vi "记录字符串解析到数组表.vi"(9 "导出条件":T1, 10 "记录数据":T9, 11 "名称":string) -> (0 "累积列表-标题行":string[](array[string])=["名称", "起始时间", "结束时间", "时长", "累积", "平均"], 1 "报警列表-标题行":string[](array[string])=["名称", "起始时间", "类型", "时长", "平均值", "最大值", "累积", "结论"], 2 "报警列表数组":string[][](array[string]), 3 "累积记录数组":string[][](array[string]))   [LabVIEW 2017]
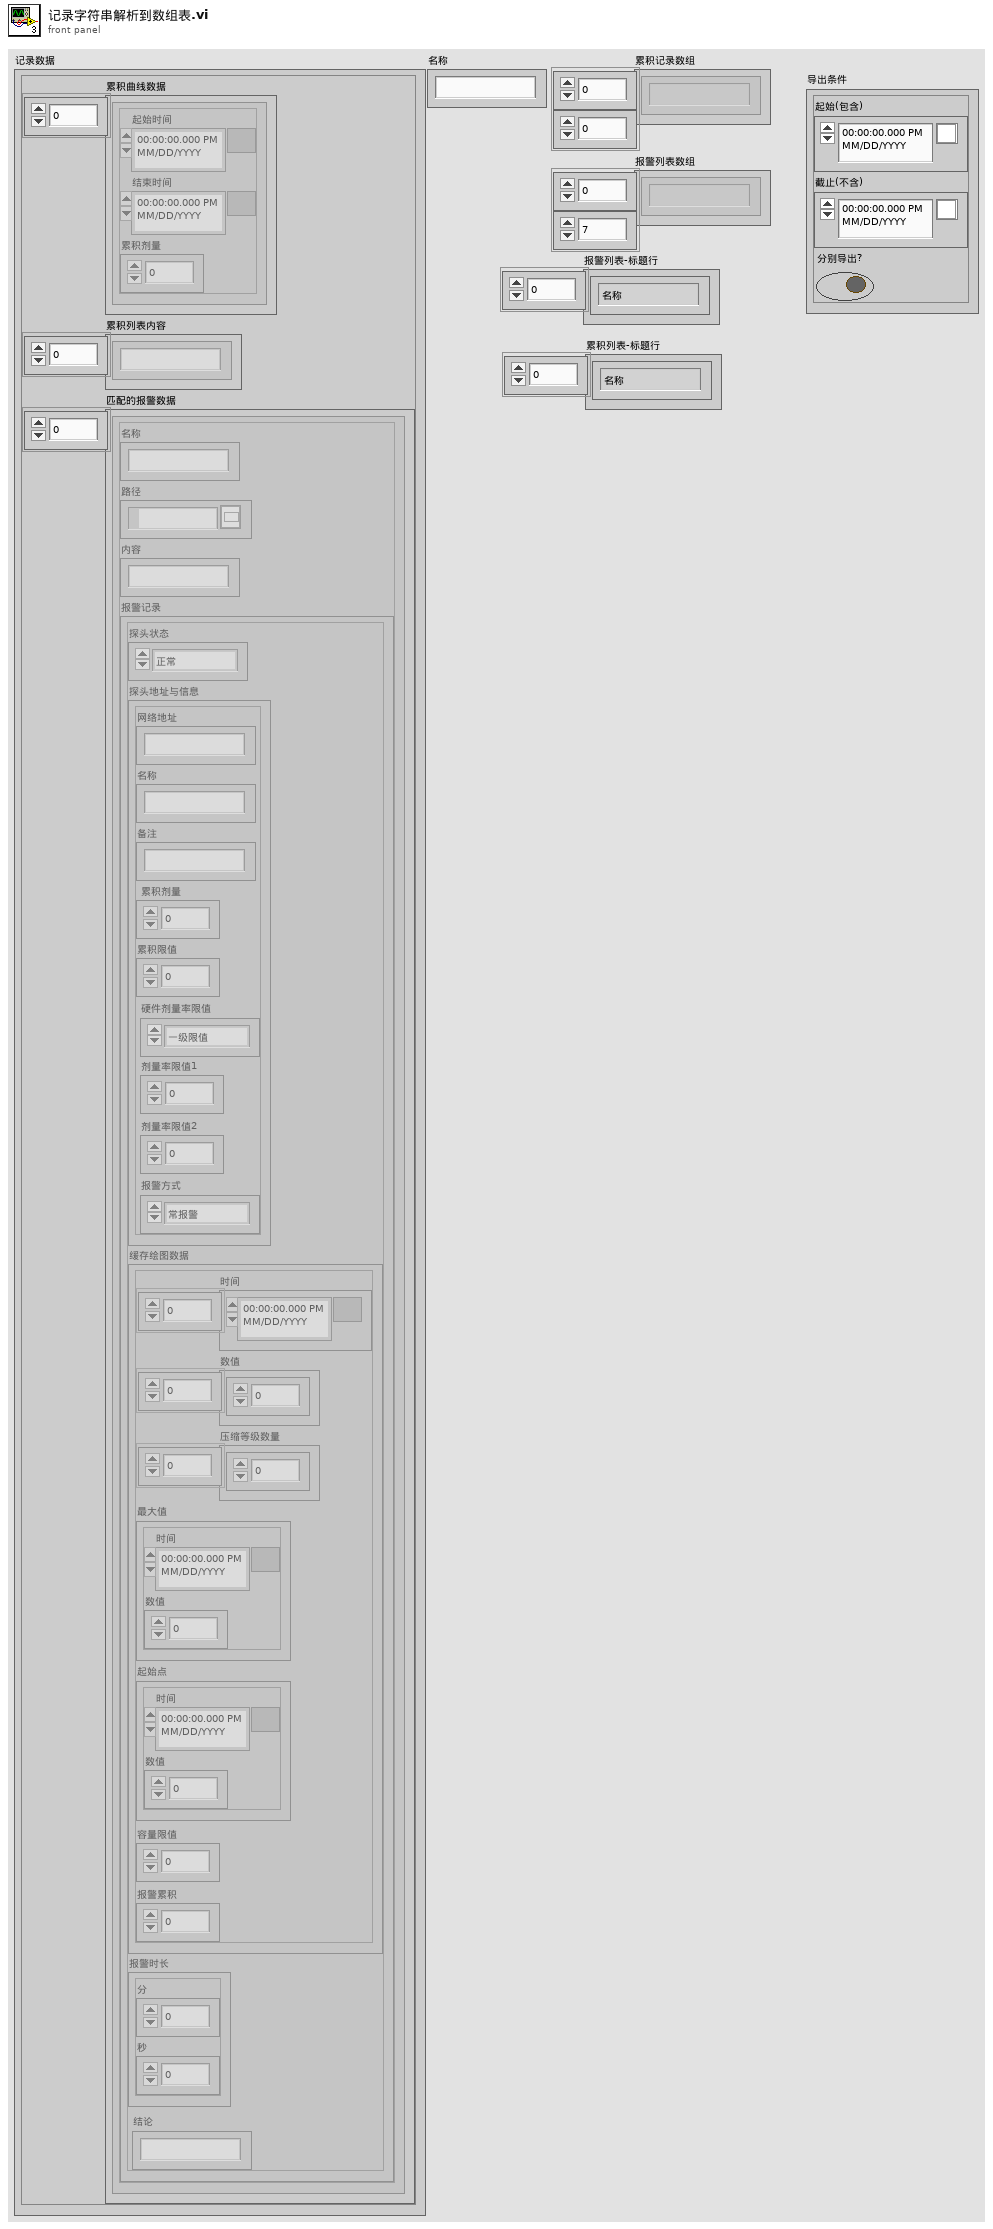
[diagram p1: front panel]
types:
  T1 = typedef "文件导出条件.ctl" = cluster{"起始(包含)":timestamp, "截止(不含)":timestamp, "分别导出?":bool}
  T2 = typedef "单条累积记录.ctl" = cluster{"起始时间":timestamp, "结束时间":timestamp, "累积剂量":dbl}
  T3 = typedef "通用报警记录.ctl" = cluster{"探头状态":T4, "探头地址与信息":T5, "缓存绘图数据":T8, "平均值":dbl, "报警时长":cluster{"分":u16, "秒":u16}, "结论":string}
  T4 = typedef "探头状态.ctl" = enum16{"正常", "离线", "禁用", "一级报警", "二级报警", "累积报警"}
  T5 = typedef "探测器信息.ctl" = cluster{"网络地址":string, "名称":string, "备注":string, "累积剂量":dbl, "累积限值":dbl, "硬件剂量率限值":T6, "剂量率限值1":dbl, "剂量率限值2":dbl, "报警方式":T7}
  T6 = typedef "探头剂量率限值选择.ctl" = enum16{"一级限值", "二级限值"}
  T7 = typedef "报警方式选择.ctl" = enum16{"常报警", "自动静音", "手动静音"}
  T8 = typedef "时值缓存压缩模块.lvlib/缓存数据.ctl" = cluster{"时间":timestamp[], "数值":dbl[], "压缩等级数量":i32[], "最大值":cluster{"时间":timestamp, "数值":dbl}, "起始点":cluster{"时间":timestamp, "数值":dbl}, "容量限值":i32, "报警累积":dbl}
  T9 = cluster{"累积曲线数据":T2[], "累积列表内容":string[], "匹配的报警数据":cluster{"名称":string, "路径":path, "内容":string, "报警记录":T3}[]}
  T10 = cluster{"名称":string, "路径":path, "内容":string, "报警记录":T3}[]
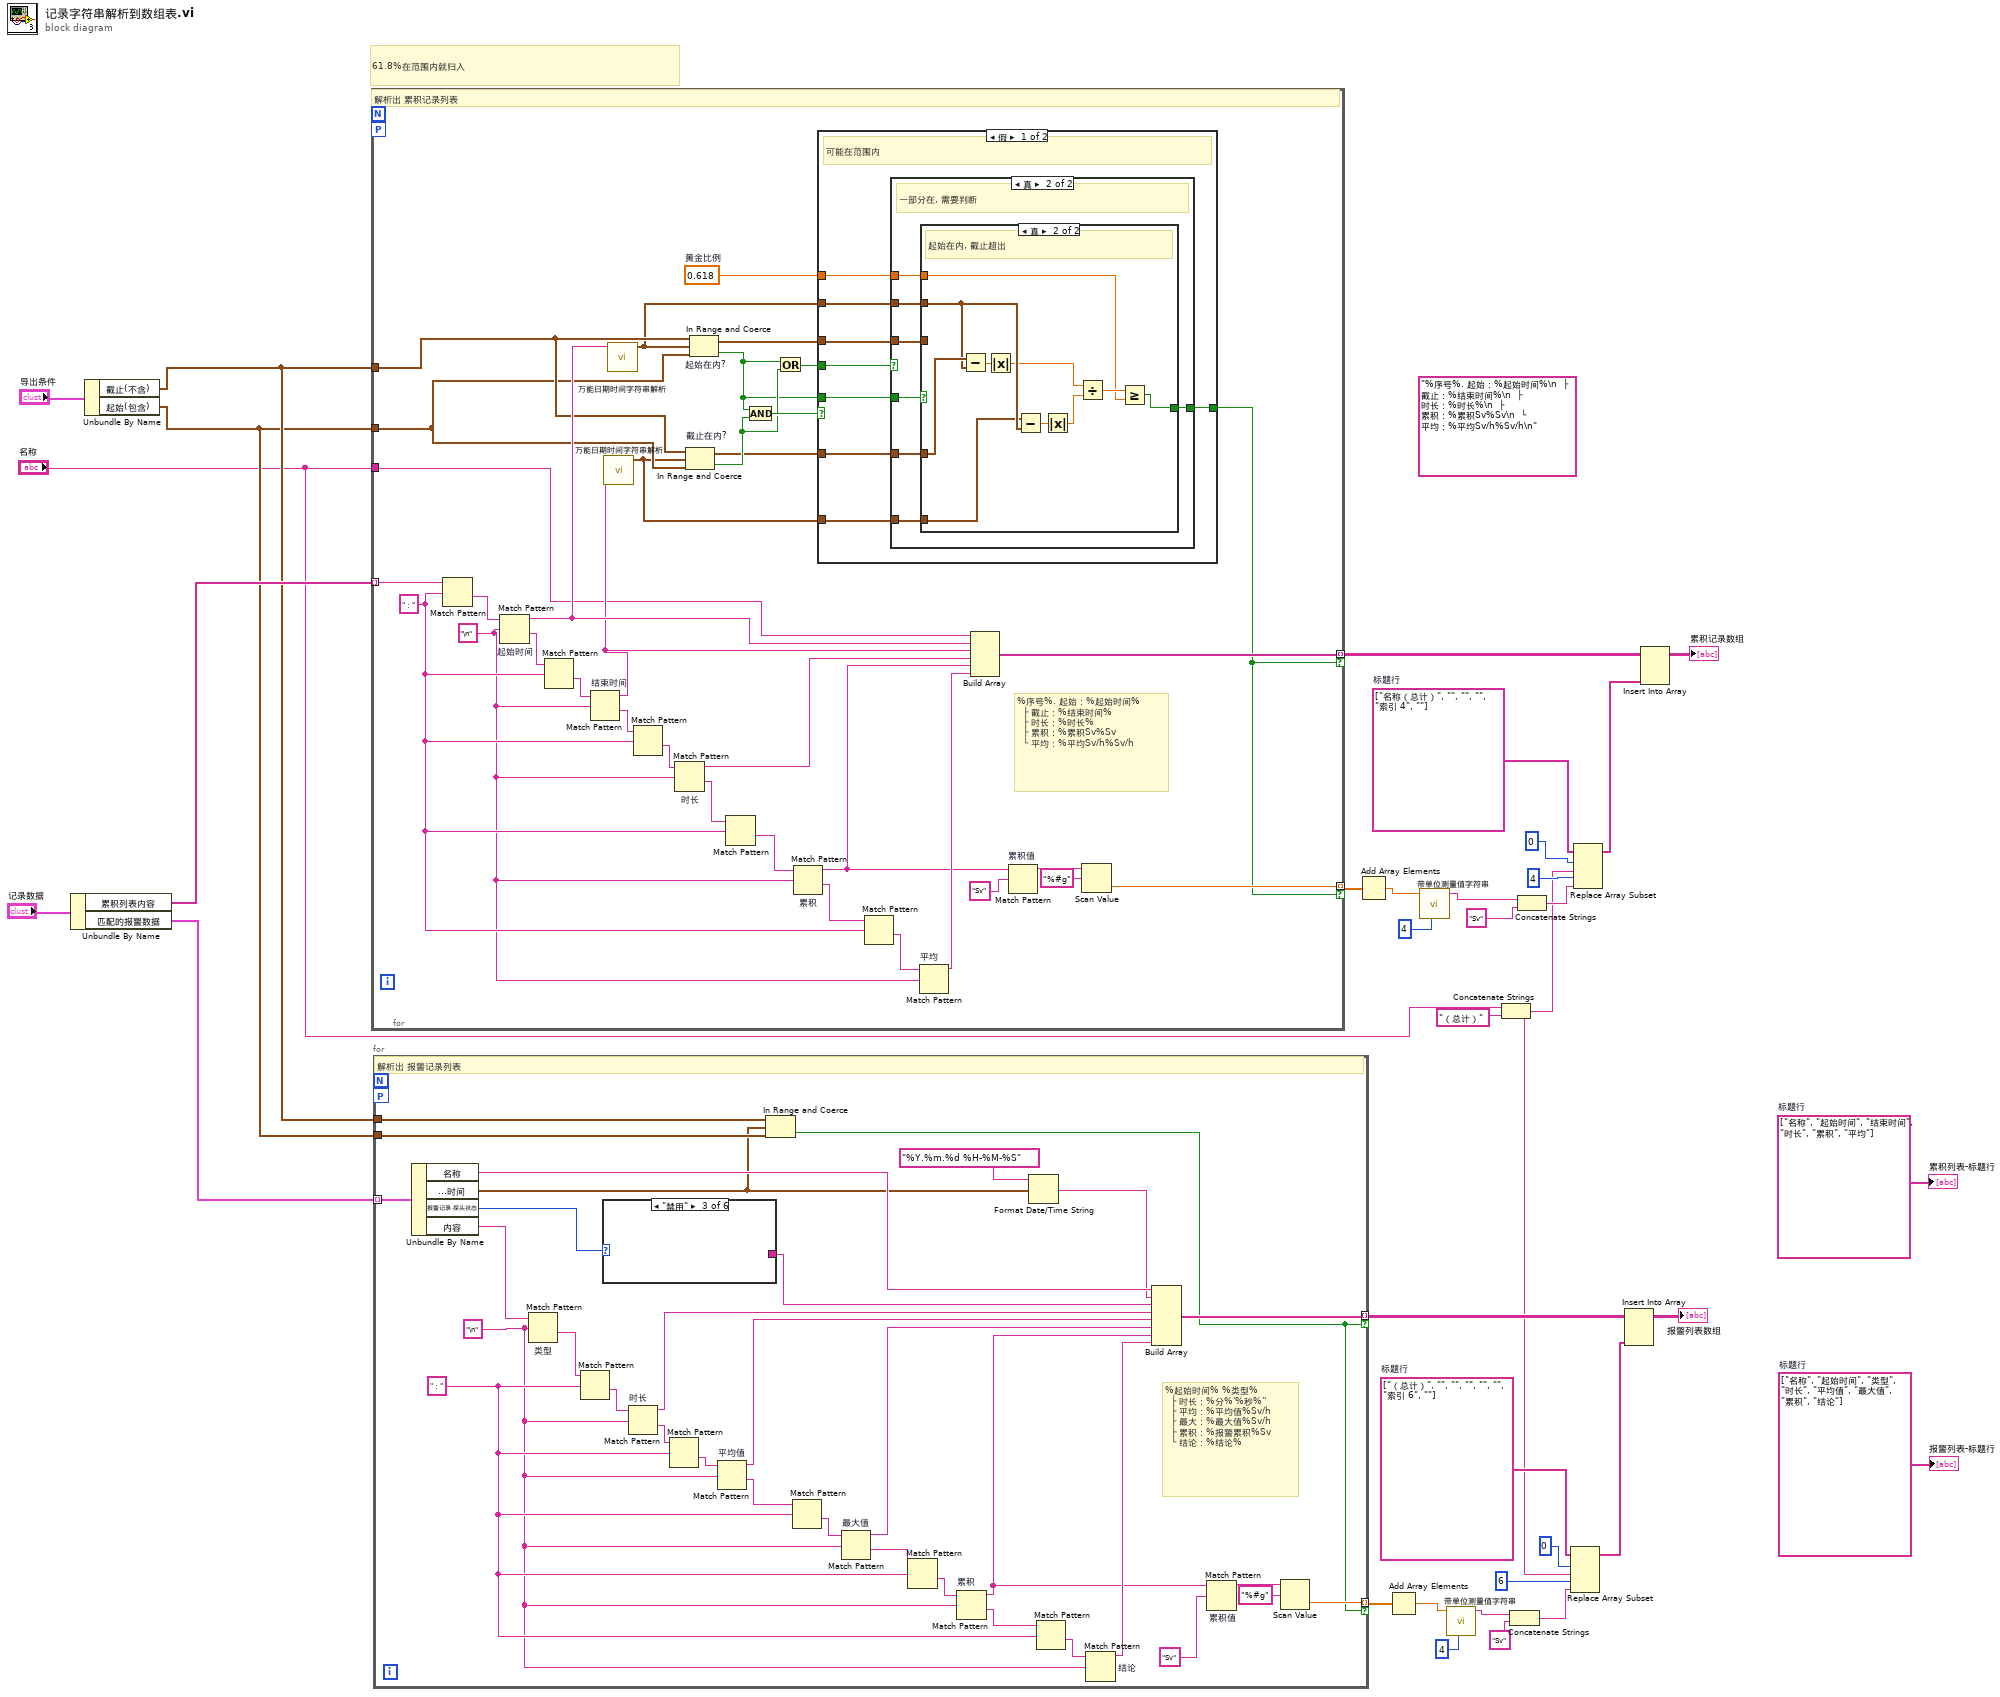
[diagram p0: block diagram]
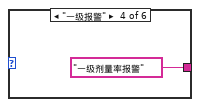
[diagram p4: hidden frame]
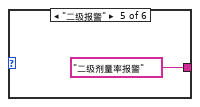
[diagram p5: hidden frame]
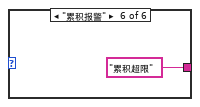
[diagram p6: hidden frame]
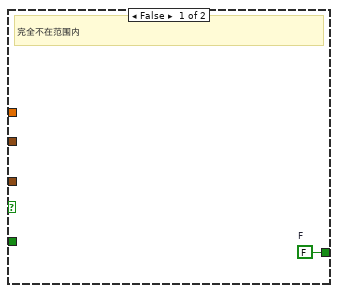
[diagram p7: hidden frame]
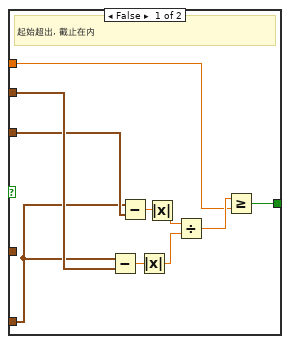
[diagram p8: hidden frame]
diagram:
  w25 = string[] ["（总计）", "", "", "", "", "", "索引 6", ""]  # 标题行
  w17 = string[] ["名称（总计）", "", "", "", "索引 4", ""]  # 标题行
  (unwired) "%序号%. 起始：%起始时间%\n  ├ 截止：%结束时间%\n  ├ 时长：%时长%\n  ├ 累积：%累积Sv%Sv\n  └ 平均：%平均Sv/h%Sv/h\n" ("Result")
  w32 = string[] ["名称", "起始时间", "类型", "时长", "平均值", "最大值", "累积", "结论"]  # 标题行
  w31 = string[] ["名称", "起始时间", "结束时间", "时长", "累积", "平均"]  # 标题行
  # "61.8%在范围内就归入"
  n1 = Unbundle By Name("记录数据") -> ("累积列表内容"=w34:string[], "匹配的报警数据"=w33:T10)
  n2 = Unbundle By Name("导出条件") -> ("截止(不含)"=w29:timestamp, "起始(包含)"=w28:timestamp)
  n3 = for {
    tunnel: w34 -> [w70] mode=indexing
    tunnel: "名称" -> [w51]
    tunnel: [w56] -> w14 mode=indexing if=w36
    tunnel: w29 -> [w53]
    tunnel: w28 -> [w52]
    workers-P: _ -> [_]
    tunnel: [w37] -> w27 mode=indexing if=w36
    w42 = 0.618  # 黄金比例
    w65 = "\n"
    w66 = "：" ("正则表达式")
    # "%序号%. 起始：%起始时间%\n  ├ 截止：%结束时间%\n  ├ 时长：%时长%\n  ├ 累积：%累积Sv%Sv\n  └ 平均：%平均Sv/h%Sv/h"
    # "解析出 累积记录列表"
    n4 = Match Pattern(string=w70, regular expression=w66) -> (after substring=w69:string)  [unwired: 1 in, 3 out]
    n5 = Match Pattern "起始时间"(string=w69, regular expression=w65) -> (before substring=w55:string, after substring=w68:string)  [unwired: 1 in, 2 out]
    n6 = Match Pattern(string=w68, regular expression=w66) -> (after substring=w67:string)  [unwired: 1 in, 3 out]
    n7 = Match Pattern "结束时间"(string=w67, regular expression=w65) -> (before substring=w54:string, after substring=w64:string)  [unwired: 1 in, 2 out]
    n8 = call "万能日期时间字符串解析.vi"("日期时间字符串"=w54) -> ("时间标识"=w46:timestamp)  [unwired: 9 in, 1 out]
    n9 = call "万能日期时间字符串解析.vi"("日期时间字符串"=w55) -> ("时间标识"=w45:timestamp)  [unwired: 9 in, 1 out]
    n10 = Match Pattern(string=w64, regular expression=w66) -> (after substring=w63:string)  [unwired: 1 in, 3 out]
    n11 = Match Pattern "时长"(string=w63, regular expression=w65) -> (before substring=w58:string, after substring=w62:string)  [unwired: 1 in, 2 out]
    n12 = In Range and Coerce "截止在内?"(upper limit=w53, x=w46, lower limit=w52) -> (coerced(x)=w43:timestamp, In Range?=w49:bool)
    n13 = In Range and Coerce "起始在内?"(upper limit=w53, x=w45, lower limit=w52) -> (coerced(x)=w44:timestamp, In Range?=w47:bool)
    n14 = Match Pattern(string=w62, regular expression=w66) -> (after substring=w61:string)  [unwired: 1 in, 3 out]
    n15 = And(x=w47, y=w49) -> (x .and. y?=w50:bool)
    n16 = Or(x=w47, y=w49) -> (x .or. y?=w48:bool)
    n17 = Match Pattern "累积"(string=w61, regular expression=w65) -> (before substring=w41:string, after substring=w60:string)  [unwired: 1 in, 2 out]
    n18 = case shown="假" w50 {
      selector: w50 -> [_ w107]
      tunnel: [w71 w107] -> w36
      tunnel: w48 -> [w78 _]
      tunnel: w47 -> [w77 _]
      tunnel: w46 -> [w76 _]
      tunnel: w45 -> [w75 _]
      tunnel: w44 -> [w74 _]
      tunnel: w43 -> [w73 _]
      tunnel: w42 -> [w72 _]
      frame False {
        # "可能在范围内"
        n19 = case shown="真" w78 {
          tunnel: w77 -> [_ w86]
          tunnel: w76 -> [_ w85]
          tunnel: w75 -> [_ w84]
          tunnel: w74 -> [_ w83]
          tunnel: w73 -> [_ w82]
          tunnel: w72 -> [_ w81]
          tunnel: [w79 w80] -> w71
          frame False {
            w79 = FALSE  # F
            # "完全不在范围内"
          }
          frame True {
            # "一部分在, 需要判断"
            n20 = case shown="真" w86 {
              tunnel: w85 -> [w91 w104]
              tunnel: w84 -> [w93 w105]
              tunnel: w83 -> [w92 _]
              tunnel: w82 -> [_ w106]
              tunnel: w81 -> [w88 w99]
              tunnel: [w87 w98] -> w80
              frame False {
                # "起始超出, 截止在内"
                n21 = Subtract(x=w91, y=w93) -> (x-y=w96:dbl)
                n22 = Subtract(x=w91, y=w92) -> (x-y=w90:dbl)
                n23 = Absolute Value(x=w96) -> (abs(x)=w95:dbl)
                n24 = Absolute Value(x=w90) -> (abs(x)=w94:dbl)
                n25 = Divide(x=w94, y=w95) -> (x/y=w89:dbl)
                n26 = Greater Or Equal?(x=w89, y=w88) -> (x >= y?=w87:bool)
              }
              frame True {
                # "起始在内, 截止超出"
                n27 = Subtract(x=w106, y=w105) -> (x-y=w97:dbl)
                n28 = Absolute Value(x=w97) -> (abs(x)=w101:dbl)
                n29 = Subtract(x=w104, y=w105) -> (x-y=w103:dbl)
                n30 = Absolute Value(x=w103) -> (abs(x)=w102:dbl)
                n31 = Divide(x=w101, y=w102) -> (x/y=w100:dbl)
                n32 = Greater Or Equal?(x=w100, y=w99) -> (x >= y?=w98:bool)
              }
            }
          }
        }
      }
      frame True {
        # "绝对在这个范围内"
      }
    }
    n33 = Match Pattern(string=w60, regular expression=w66) -> (after substring=w59:string)  [unwired: 1 in, 3 out]
    n34 = Match Pattern "平均"(string=w59, regular expression=w65) -> (before substring=w57:string)  [unwired: 1 in, 3 out]
    n35 = Build Array(w51, w55, w54, w58, w41, w57) -> (w56:string[])
    n36 = Match Pattern "累积值"(string=w41, regular expression="Sv" ("正则表达式")) -> (before substring=w39:string)  [unwired: 1 in, 3 out]
    n37 = Scan Value(string=w39, format string="%#g" ("格式字符串")) -> (value=w37:dbl)  [unwired: 1 in, 1 out]
  }
  n38 = for {
    tunnel: w33 -> [w140] mode=indexing
    tunnel: [w122] -> w21 mode=indexing if=w114
    tunnel: w29 -> [w121]
    tunnel: w28 -> [w120]
    tunnel: [w115] -> w26 mode=indexing if=w114
    workers-P: _ -> [_]
    w137 = "：" ("正则表达式")
    w136 = "\n"
    # "%起始时间% %类型%\n  ├ 时长：%分%'%秒%''\n  ├ 平均：%平均值%Sv/h\n  ├ 最大：%最大值%Sv/h\n  ├ 累积：%报警累积%Sv\n  └ 结论：%结论%"
    # "解析出 报警记录列表"
    n39 = Unbundle By Name(w140) -> ("名称"=w139:string, "报警记录.缓存绘图数据.起始点.时间"=w111:timestamp, "报警记录.探头状态"=w110:T4, "内容"=w108:string)
    n40 = Match Pattern "类型"(string=w108, regular expression=w136) -> (after substring=w138:string)  [unwired: 1 in, 3 out]
    n41 = Match Pattern(string=w138, regular expression=w137) -> (after substring=w135:string)  [unwired: 1 in, 3 out]
    n42 = case shown="\"禁用\"" w110 {
      tunnel: [_ _ _ "一级剂量率报警" "二级剂量率报警" "累积超限"] -> w109
      frame "正常", Default {
      }
      frame "离线" {
      }
      frame "禁用" {
      }
      frame "一级报警" {
      }
      frame "二级报警" {
      }
      frame "累积报警" {
      }
    }
    n43 = Match Pattern "时长"(string=w135, regular expression=w136) -> (before substring=w126:string, after substring=w134:string)  [unwired: 1 in, 2 out]
    n44 = Match Pattern(string=w134, regular expression=w137) -> (after substring=w133:string)  [unwired: 1 in, 3 out]
    n45 = Match Pattern "平均值"(string=w133, regular expression=w136) -> (before substring=w125:string, after substring=w132:string)  [unwired: 1 in, 2 out]
    n46 = In Range and Coerce(upper limit=w121, x=w111, lower limit=w120) -> (In Range?=w114:bool)  [unwired: 1 out]
    n47 = Match Pattern(string=w132, regular expression=w137) -> (after substring=w131:string)  [unwired: 1 in, 3 out]
    n48 = Match Pattern "最大值"(string=w131, regular expression=w136) -> (before substring=w124:string, after substring=w130:string)  [unwired: 1 in, 2 out]
    n49 = Match Pattern(string=w130, regular expression=w137) -> (after substring=w129:string)  [unwired: 1 in, 3 out]
    n50 = Match Pattern "累积"(string=w129, regular expression=w136) -> (before substring=w116:string, after substring=w128:string)  [unwired: 1 in, 2 out]
    n51 = Format Date/Time String(time format string (%c)="%Y.%m.%d %H-%M-%S" ("时间格式字符串(%c)"), seconds (now)=w111) -> (date/time string=w112:string)  [unwired: 1 in]
    n52 = Match Pattern(string=w128, regular expression=w137) -> (after substring=w127:string)  [unwired: 1 in, 3 out]
    n53 = Match Pattern "结论"(string=w127, regular expression=w136) -> (before substring=w123:string)  [unwired: 1 in, 3 out]
    n54 = Build Array(w139, w112, w109, w126, w125, w124, w116, w123) -> (w122:string[])
    n55 = Match Pattern "累积值"(string=w116, regular expression="Sv" ("正则表达式")) -> (before substring=w118:string)  [unwired: 1 in, 3 out]
    n56 = Scan Value(string=w118, format string="%#g" ("格式字符串")) -> (value=w115:dbl)  [unwired: 1 in, 1 out]
  }
  n57 = Add Array Elements(numeric array=w27) -> (sum=w11:dbl)
  n58 = Add Array Elements(numeric array=w26) -> (sum=w8:dbl)
  n59 = call "带单位测量值字符串.vi"("精度(2)"=i16 4, "测量值"=w11) -> ("结果"=w10:string)  [unwired: 9 in]
  n60 = call "带单位测量值字符串.vi"("精度(2)"=i16 4, "测量值"=w8) -> ("结果"=w6:string)  [unwired: 9 in]
  n61 = Concatenate Strings("名称", "（总计）" ("正则表达式")) -> (w1:string)
  n62 = Concatenate Strings(w6, "Sv" ("正则表达式")) -> (w23:string)
  n63 = Concatenate Strings(w10, "Sv" ("正则表达式")) -> (w18:string)
  n64 = Replace Array Subset(array=w25, new element #1=w1, index #1=0 ("索引"), new element #2=w23, index #2=6 ("索引")) -> (w20:string[])
  n65 = Replace Array Subset(array=w17, new element #1=w1, index #1=0 ("索引"), new element #2=w18, index #2=4 ("索引")) -> (w15:string[])
  n66 = Insert Into Array(array=w21, new element=w20) -> (→"报警列表数组":string[][])  [unwired: 2 in]
  n67 = Insert Into Array(array=w14, new element=w15) -> (→"累积记录数组":string[][])  [unwired: 2 in]
  "报警列表-标题行" <- w32
  "累积列表-标题行" <- w31
